vi "output.vi"(3 "error in (no error)":errorcluster, 4 "Tuner":dbl, 5 "commando":string, 6 "VISA in":refnum<visa-resource-name>) -> (0 "error out":errorcluster, 1 "Output":string, 2 "VISA out":refnum<visa-resource-name>)   [LabVIEW 2019]
uses:
  <vilib>/Instr/_visa.llb/VISA Configure Serial Port (Instr).vi
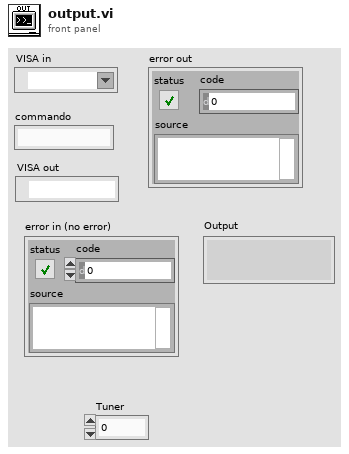
[diagram p1: front panel]
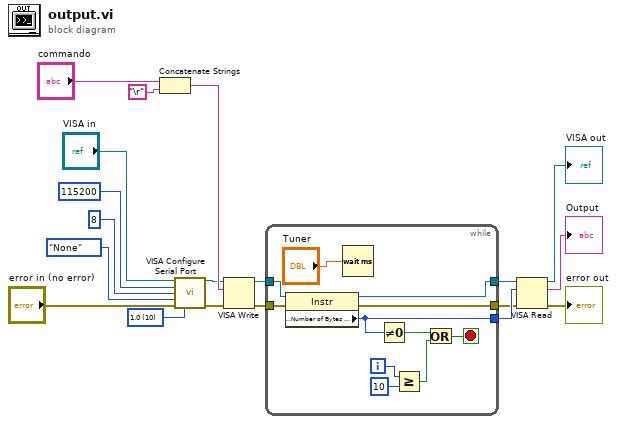
[diagram p0: block diagram]
diagram:
  w19 = u16 10 items=["1.0"=10, "1.5"=15, "2.0"=20] ("stop bits (10: 1 bit)")
  n1 = Concatenate Strings("commando", "\r") -> (w17:string)
  n2 = call-poly "VISA Configure Serial Port"("VISA resource name"="VISA in", "baud rate (9600)"=u32 115200, "data bits (8)"=u16 8, "parity (0:none)"=enum16{"None", "Odd", "Even", "Mark", "Space"}."None", "error in (no error)"="error in (no error)", "stop bits (10: 1 bit)"=w19) -> ("VISA resource name out"=w12:refnum<visa-resource-name>, "error out"=w13:errorcluster)  [unwired: 8 in]
  n3 = VISA Write(VISA resource name=w12, write buffer=w17, error in (no error)=w13) -> (VISA resource name out=w6:refnum<visa-resource-name>, error out=w3:errorcluster)  [unwired: 1 out]
  n4 = while {
    tunnel: w6 -> [w25]
    tunnel: [w24] -> w5
    tunnel: [w23] -> w4
    tunnel: w3 -> [w22]
    tunnel: [w21] -> w2
    i -> [w30]
    stop <- w28 stop-if-true
    n5 = property class="Instr"(reference=w25, error in=w22) -> (reference out=w24:refnum<visa-resource-name>, error out=w21:errorcluster, "Serial Settings:Number of Bytes at Serial Port"=w23:u32)
    n6 = Wait (ms)(milliseconds to wait="Tuner") -> ()  [unwired: 1 out]
    n7 = Not Equal To 0?(x=w23) -> (x != 0?=w26:bool)
    n8 = Greater Or Equal?(x=w30, y=10) -> (x >= y?=w27:bool)
    n9 = Or(x=w26, y=w27) -> (x .or. y?=w28:bool)
  }
  n10 = VISA Read(VISA resource name=w5, byte count=w4, error in (no error)=w2) -> (VISA resource name out=→"VISA out":refnum<visa-resource-name>, read buffer=→"Output":string, error out=→"error out":errorcluster)  [unwired: 1 out]
